vi "Get Resource ID.vi"(4 "I2C in":refnum<class "I2C.lvclass">) -> (7 "Resource ID":string)   [LabVIEW 2020, in "CTI.lvlib" / "I2C.lvclass"]
uses:
  I2C.lvclass
  I2C.lvclass/I2C.ctl
  GPIO/GPIO.lvclass/GPIO.ctl
  GPIO/GPIO.lvclass
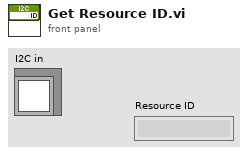
[diagram p1: front panel]
types:
  T1 = typedef "CTI.lvlib/I2C Number.ctl" = i8
  T2 = typedef "CTI.lvlib/GPIO Number.ctl" = i8
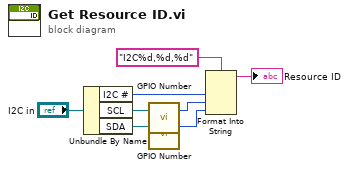
[diagram p0: block diagram]
diagram:
  n1 = Unbundle By Name("I2C in") -> ("I2C #"=w4:T1, "SCL"=w6:refnum<class "GPIO.lvclass">, "SDA"=w5:refnum<class "GPIO.lvclass">)
  n2 = call "GPIO Number.vi"("GPIO in"=w6) -> ("GPIO #"=w3:T2)  [unwired: 6 in]
  n3 = call "GPIO Number.vi"("GPIO in"=w5) -> ("GPIO #"=w2:T2)  [unwired: 6 in]
  n4 = Format Into String(format string="I2C%d,%d,%d", w4, w3, w2) -> (resulting string=→"Resource ID":string)  [unwired: 2 in, 1 out]
